vi "GetFeaturesToRegister.vi"(7 "high rate":bool, 8 "error in (no error)":errorcluster, 10 "group":string, 11 "channels":T1[](array[typedef])) -> (0 "error out":errorcluster, 2 "atleast one":bool, 3 "register trend":T5)   [LabVIEW 2017, in "McsaAnalysisLowRate.lvlib"]
uses:
  <vilib>/addons/InsightCM/Devices/Shared/Mcsa/McsaAnalysisLowRate/McsaAnalysisLowRate.lvlib
  <vilib>/addons/InsightCM/Devices/Shared/Common/DataEventCreator/controls/RegisterTrendPoints.ctl
  <vilib>/addons/InsightCM/Devices/Shared/Common/DataEventCreator/controls/Registry_Trend.ctl
  <vilib>/addons/InsightCM/Utilities/Analysis/MCSA/controls/McsaChannel.ctl
  <vilib>/addons/InsightCM/Utilities/Analysis/Shared/controls/Feature.ctl
  <vilib>/addons/InsightCM/Utilities/Analysis/Shared/controls/AmplitudeScale.ctl
  <vilib>/addons/InsightCM/MessageBus/Base/controls/KeyValuePair.ctl
  <vilib>/addons/InsightCM/Devices/Shared/Common/DataEventCreator/DataEventCreator.lvlib
  <vilib>/addons/InsightCM/Utilities/Analysis/Shared/AnalysisHelper.lvlib
  <vilib>/addons/InsightCM/Utilities/Analysis/MCSA/McsaAnalysisFunctions.lvlib
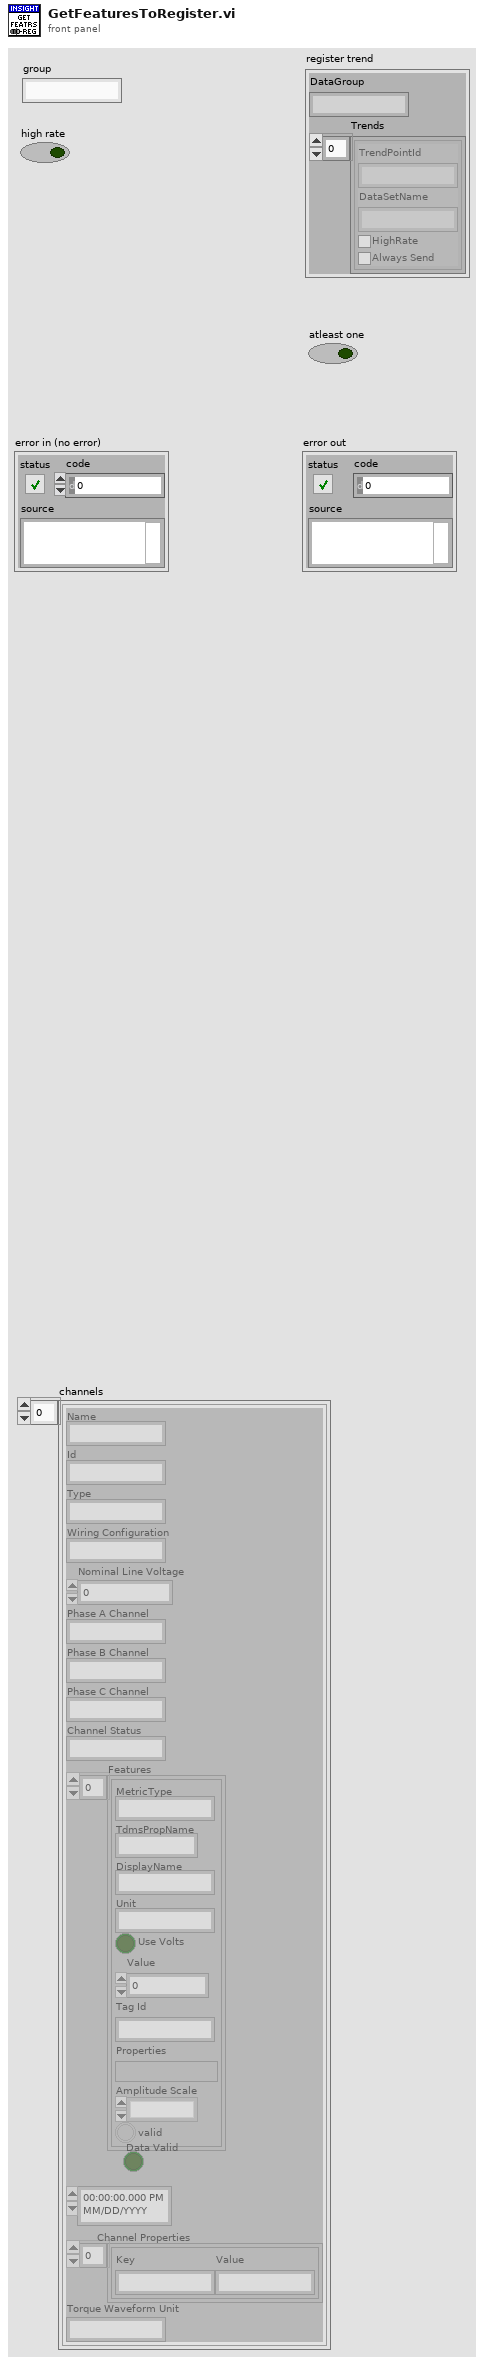
[diagram p1: front panel]
types:
  T1 = typedef "McsaAnalysisFunctions.lvlib/McsaChannel.ctl" = cluster{"Name":string, "Id":string, "Type":string, "Wiring Configuration":string, "Nominal Line Voltage":dbl, "Phase A Channel":string, "Phase B Channel":string, "Phase C Channel":string, "Channel Status":string, "Features":T2[], "Data Valid":bool, "Acq Timestamp":timestamp, "Channel Properties":T4[], "Torque Waveform Unit":string}
  T2 = typedef "AnalysisHelper.lvlib/Feature.ctl" = cluster{"MetricType":string, "TdmsPropName":string, "DisplayName":string, "Unit":string, "Use Volts":bool, "Value":dbl, "Tag Id":string, "Properties":variant, "Amplitude Scale":T3, "valid":bool}
  T3 = typedef "AnalysisHelper.lvlib/AmplitudeScale.ctl" = enum16{"rms", "peak", "pk-pk"}
  T4 = typedef "KeyValuePair.ctl" = cluster{"Key":string, "Value":string}
  T5 = typedef "DataEventCreator.lvlib/RegisterTrendPoints.ctl" = cluster{"DataGroup":string, "Trends":T6[]}
  T6 = typedef "DataEventCreator.lvlib/Registry_Trend.ctl" = cluster{"TrendPointId":string, "DataSetName":string, "HighRate":bool, "Always Send":bool}
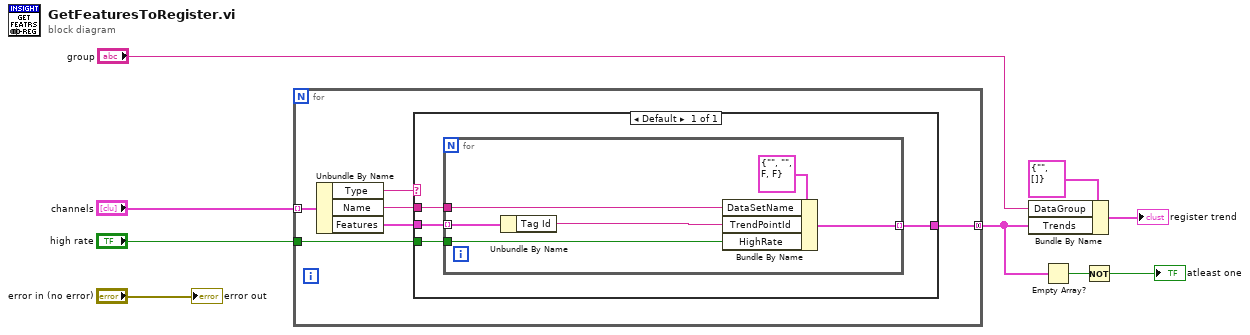
[diagram p0: block diagram]
diagram:
  n1 = for {
    tunnel: "channels" -> [w15] mode=indexing
    tunnel: [w13] -> w5 mode=concatenating
    tunnel: "high rate" -> [w10]
    n2 = Unbundle By Name(w15) -> ("Type"=w11:string, "Name"=w12:string, "Features"=w14:T2[])
    n3 = case shown="Default" w11 {
      tunnel: w14 -> [w19]
      tunnel: [w18] -> w13
      tunnel: w12 -> [w17]
      tunnel: w10 -> [w16]
      frame Default {
        n4 = for {
          tunnel: w19 -> [w20] mode=indexing
          tunnel: [w25] -> w18 mode=indexing
          tunnel: w17 -> [w24]
          tunnel: w16 -> [w21]
          n5 = Unbundle By Name(w20) -> ("Tag Id"=w23:string)
          n6 = Bundle By Name(cluster=T6 {"TrendPointId"="", "DataSetName"="", "HighRate"=FALSE, "Always Send"=FALSE} ("Trend"), "DataSetName"=w24, "TrendPointId"=w23, "HighRate"=w21) -> (w25:T6)
        }
      }
    }
  }
  n7 = Bundle By Name(cluster=T5 {"DataGroup"="", "Trends"=[]} ("RegisterTrend"), "DataGroup"="group", "Trends"=w5) -> (→"register trend":T5)
  n8 = Empty Array?(array=w5) -> (empty?=w6:bool)
  n9 = Not(x=w6) -> (.not. x?=→"atleast one":bool)
  "error out" <- "error in (no error)"
